vi "data setup.vi"(0 "Serial Port":refnum<visa-resource-name>, 5 "data rate":T1(ring)=enum."10 Hz") -> (4 "Serial Port":refnum<visa-resource-name>, 6 "data points":u8, 8 "delta x":dbl format="%.4f")   [LabVIEW 2012]
panel:
  in  "signals":enum16{"signal 1", "signals 1 and 2"}(ring)
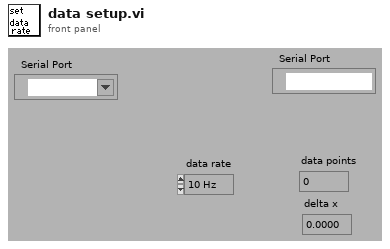
[diagram p1: front panel]
types:
  T1 = enum16{"20 Hz", "10 Hz", "5 Hz", "2.5 Hz", "1.25 Hz"}
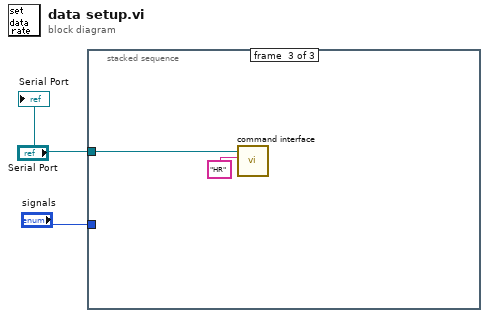
[diagram p0: block diagram]
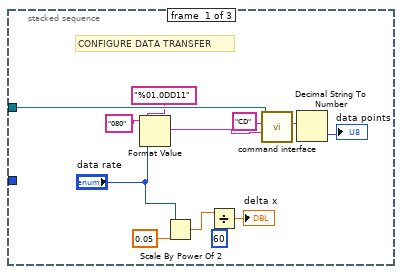
[diagram p2: hidden frame]
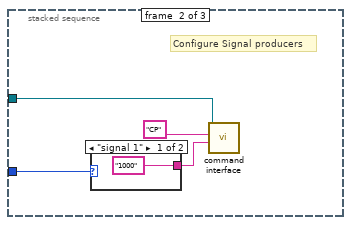
[diagram p3: hidden frame]
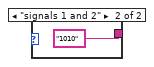
[diagram p4: hidden frame]
diagram:
  n1 = stacked-sequence {
    tunnel: "Serial Port" -> [w14 w18 w21]
    tunnel: "signals" -> [_ w15 _]
    frame #0 {
      # "CONFIGURE DATA TRANSFER"
      n2 = Format Value(string ("")="080", format string="%01.0DD11", value (0)="data rate") -> (output string=w9:string)
      n3 = Scale By Power Of 2(n="data rate", x=0.05) -> (x*2^n=w6:dbl)
      n4 = Divide(x=w6, y=60) -> (x/y=→"delta x":dbl)
      n5 = call "command interface.vi"("Parameter"=w9, "command"="CD", "Serial Port"=w14) -> ("response"=w12:string)  [unwired: 4 in, 3 out]
      n6 = Decimal String To Number(string=w12) -> (number=→"data points":i32)  [unwired: 2 in, 1 out]
    }
    frame #1 {
      # "Configure Signal producers"
      n7 = case shown="\"signal 1\"" w15 {
        tunnel: ["1000" "1010"] -> w16
        frame "signal 1" {
        }
        frame "signals 1 and 2" {
        }
      }
      n8 = call "command interface.vi"("Parameter"=w16, "command"="CP", "Serial Port"=w18) -> ()  [unwired: 4 in, 4 out]
    }
    frame #2 {
      n9 = call "command interface.vi"("command"="HR", "Serial Port"=w21) -> ()  [unwired: 5 in, 4 out]
    }
  }
  "Serial Port" <- "Serial Port"
